vi "handlePostRequest_changeServoParameters.vi"(12 "LabVIEW Web Service Request":refnum<class "Web Request.lvclass">) -> (1 "Position (degrees)":dbl format="%#_3g", 2 "Status":string, 13 "Message":string)   [LabVIEW 2024]
uses:
  <vilib>/wsapi/Web Request.lvclass
  <vilib>/Instr/_visa.llb/VISA Configure Serial Port (Instr).vi
panel:
  out "ESP32_out_auto":string
  out "ESP32_out_manual":string
  # "Use the Web Service Request input terminal to call the VIs on the Web Services palette. Do not remove it from the connector pane unless you don't need access to the palette."
  # "Each additional control wired to the connector pane will be available as an input in the URL. To include an indicator in terminal-mode output (the default setting), it must also be wired to the connector pane."
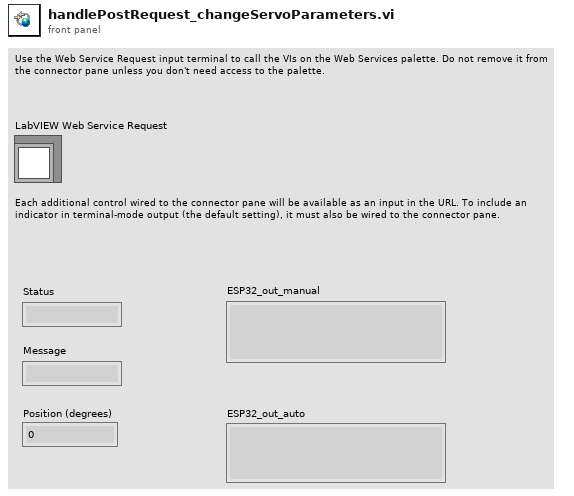
[diagram p1: front panel]
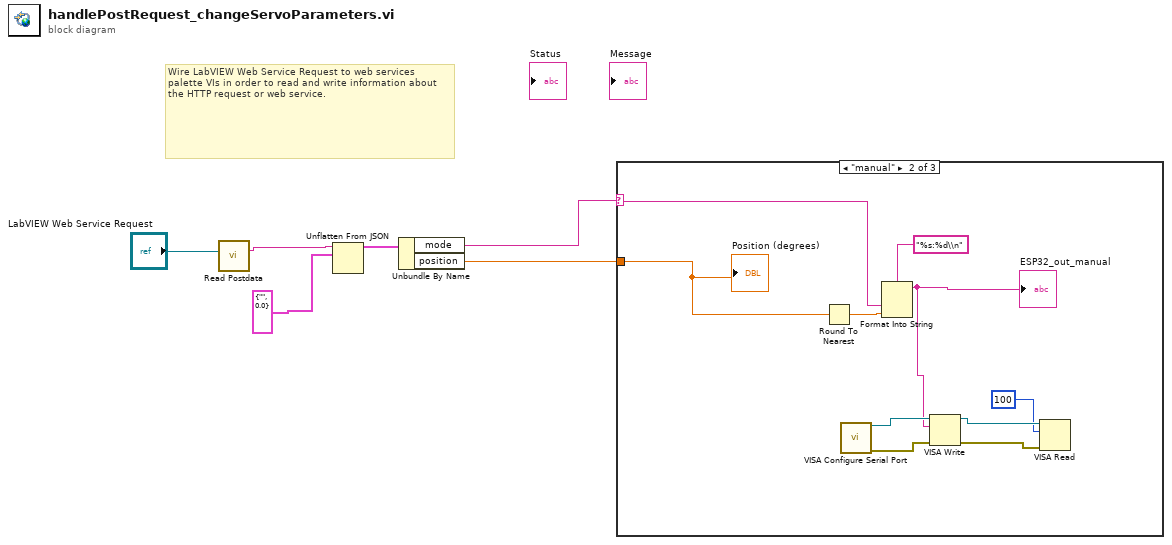
[diagram p0: block diagram]
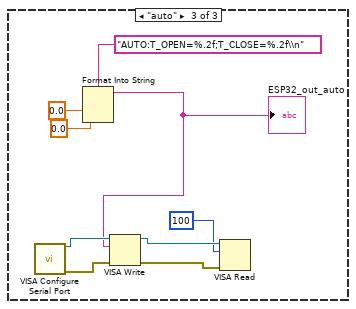
[diagram p3: hidden frame]
diagram:
  # "Wire LabVIEW Web Service Request to web services palette VIs in order to read and write information about the HTTP request or web service."
  n1 = call <vilib>:"Read Postdata.vi"("LabVIEW Web Service Request"="LabVIEW Web Service Request") -> ("postdata"=w5:string)  [unwired: 12 in, 2 out]
  n2 = Unflatten From JSON(JSON string=w5, type and defaults=cluster{"mode":string, "position":dbl} {"mode"="", "position"=0.0} ("Cluster")) -> (value=w4:cluster{"mode":string, "position":dbl})  [unwired: 5 in, 1 out]
  n3 = Unbundle By Name "Unbundle By Name"(w4) -> ("mode"=w2:string, "position"=w3:dbl)
  n4 = case shown="\"manual\"" w2 {
    selector: w2 -> [_ w11 _]
    tunnel: w3 -> [_ w10 _]
    frame "False", Default {
    }
    frame "manual" {
      n5 = Round To Nearest(number=w10) -> (nearest integer value=w9:dbl)
      n6 = call-poly "VISA Configure Serial Port"() -> ("VISA resource name out"=w15:refnum<visa-resource-name>, "error out"=w16:errorcluster)  [unwired: 14 in]
      n7 = Format Into String(format string="%s:%d\\n", w11, w9) -> (resulting string=w8:string)  [unwired: 2 in, 1 out]
      "ESP32_out_manual" <- w8
      n8 = VISA Write(VISA resource name=w15, write buffer=w8, error in (no error)=w16) -> (VISA resource name out=w13:refnum<visa-resource-name>, error out=w14:errorcluster)  [unwired: 1 out]
      n9 = VISA Read(VISA resource name=w13, byte count=100, error in (no error)=w14) -> ()  [unwired: 4 out]
      "Position (degrees)" <- w10
    }
    frame "auto" {
      n10 = call-poly "VISA Configure Serial Port"() -> ("VISA resource name out"=w24:refnum<visa-resource-name>, "error out"=w25:errorcluster)  [unwired: 14 in]
      n11 = Format Into String(format string="AUTO:T_OPEN=%.2f;T_CLOSE=%.2f\\n", 0.0 ("input 1"), 0.0 ("input 2")) -> (resulting string=w20:string)  [unwired: 2 in, 1 out]
      "ESP32_out_auto" <- w20
      n12 = VISA Write(VISA resource name=w24, write buffer=w20, error in (no error)=w25) -> (VISA resource name out=w22:refnum<visa-resource-name>, error out=w23:errorcluster)  [unwired: 1 out]
      n13 = VISA Read(VISA resource name=w22, byte count=100, error in (no error)=w23) -> ()  [unwired: 4 out]
    }
  }
